vi "AB_Engine_Package_PackedLib.vi"(5 "processed_sourceItems":T1, 7 "application package path":path, 8 "error in (no error)":errorcluster, 10 "destinations":refnum<class "AB_Destination.lvclass">[](array[class]), 11 "internal directory":path) -> (0 "error out":errorcluster, 2 "support dir":path, 3 "dup internal directory":path)   [LabVIEW 2020]
uses:
  <vilib>/AppBuilder/AB_Classes/Destination/AB_Destination.lvclass
  <vilib>/AppBuilder/AB_CopyFiles_Data.ctl
  <vilib>/AppBuilder/AB_Classes/Source/AB_Source_Processed_Info.ctl
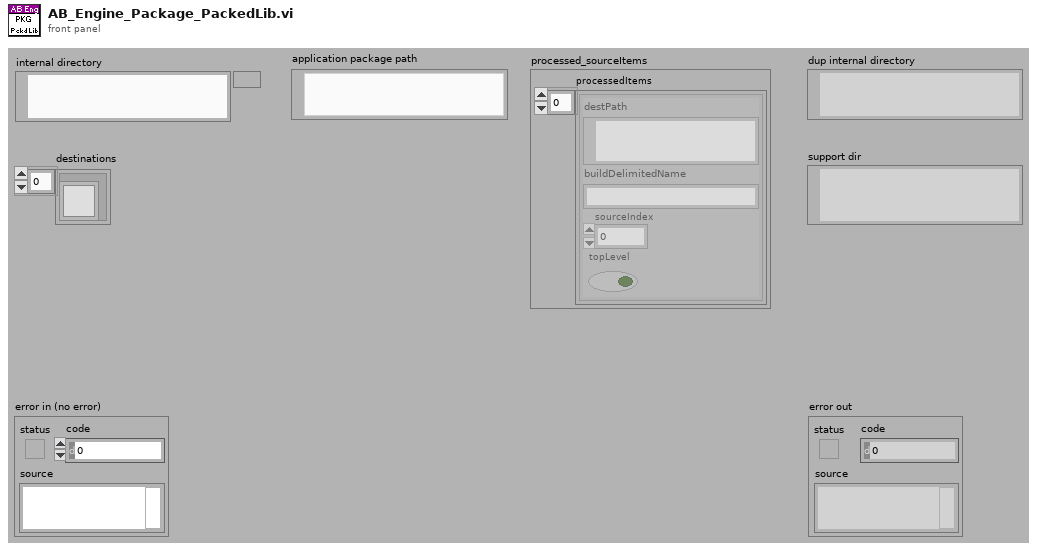
[diagram p1: front panel]
types:
  T1 = typedef "AB_CopyFiles_Data.ctl" = cluster{"processedItems":T2[]}
  T2 = typedef "AB_Source_Processed_Info.ctl" = cluster{"destPath":path, "buildDelimitedName":string, "sourceIndex":i32, "topLevel":bool}
  T3 = enum32{"invalid OS target", "Mac OS", "Windows 3.1", "Windows 95/NT", "Solaris 1", "Solaris 2", "HP-UX", "PowerMAX", "Linux", "Irix", "Rhapsody", "BeOS", "AIX", "OSF1", "VxWorks", "PharLap", "Carbon", "RTX", "Windows x64", "Linux x64", "Mac OS X x64"}
  T4 = typedef "AB_Destination.ctl" = cluster{"destName":string, "path":path, "libraryName":string, "preserveHierarchy":bool, "eng_inBuild":bool, "eng_libraryReference":refnum<vi>, "eng_restictAddToNewLibrary":bool}
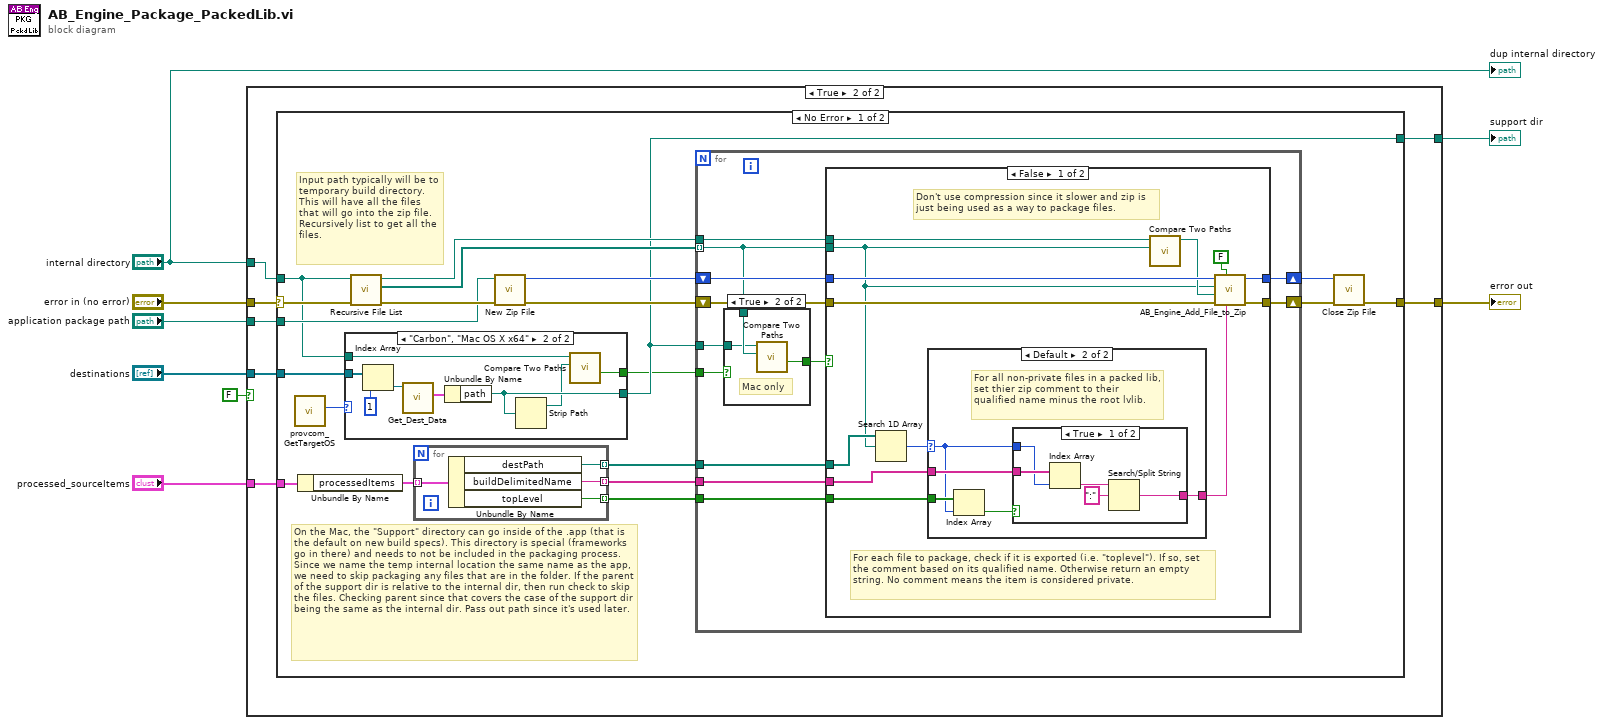
[diagram p0: block diagram]
diagram:
  n1 = case shown="True" FALSE {
    tunnel: [w9 w16] -> w8
    tunnel: "internal directory" -> [_ w15]
    tunnel: "application package path" -> [_ w14]
    tunnel: "error in (no error)" -> [w9 w13]
    tunnel: "destinations" -> [_ w12]
    tunnel: [_ w11] -> w4
    tunnel: "processed_sourceItems" -> [_ w10]
    frame False {
    }
    frame True {
      n2 = case shown="No Error" w13 {
        selector: w13 -> [w27 w89]
        tunnel: [w36 w89] -> w16
        tunnel: w15 -> [w22 _]
        tunnel: w14 -> [w28 _]
        tunnel: w12 -> [w24 _]
        tunnel: [w25 _] -> w11
        tunnel: w10 -> [w20 _]
        frame No Error {
          # "On the Mac, the \"Support\" directory can go inside of the .app (that is the default on new build specs). This directory is special (frameworks go in there) and needs to not be included in the packaging process. Since we name the temp internal location the same name as the app, we need to skip packaging any files that are in the folder. If the parent of the support dir is relative to the internal dir, then run check to skip the files. Checking parent since that covers the case of the support dir being the same as the internal dir. Pass out path since it's used later."
          # "Input path typically will be to temporary build directory. This will have all the files that will go into the zip file. Recursively list to get all the files."
          n3 = call <resource>:"provcom_GetTargetOS.vi"() -> ("App.TargetOS"=w23:T3)  [unwired: 11 out]
          n4 = Unbundle By Name(w20) -> ("processedItems"=w19:T2[])
          n5 = case shown="\"Carbon\", \"Mac OS X x64\"" w23 {
            tunnel: w24 -> [_ w41]
            tunnel: [_ w40] -> w25
            tunnel: w22 -> [_ w39]
            tunnel: [_ w37] -> w21
            frame Default {
            }
            frame "Carbon", "Mac OS X x64" {
              n6 = Index Array(array=w41, index=1) -> (element=w44:refnum<class "AB_Destination.lvclass">)
              n7 = call <vilib>:"Get_Dest_Data.vi"("Class in"=w44) -> ("destName"=w43:T4)  [unwired: 1 in, 9 out]
              n8 = Unbundle By Name(w43) -> ("path"=w40:path)
              n9 = Strip Path(path=w40) -> (stripped path=w38:path)  [unwired: 1 out]
              n10 = call <vilib>:"Compare Two Paths.vi"("Path 2"=w38, "Path 1"=w39) -> ("Path 2 Relative to Path 1?"=w37:bool)  [unwired: 1 in, 8 out]
            }
          }
          n11 = call <vilib>:"Recursive File List.vi"("error in (no error)"=w27, "Folder Path"=w22) -> ("error out"=w29:errorcluster, "All Files in Dir"=w31:path[], "dup Folder Path"=w30:path)  [unwired: 1 in, 6 out]
          n12 = for {
            tunnel: [w46] -> w26 mode=indexing
            tunnel: w19 -> [w48] mode=indexing
            tunnel: [w47] -> w18 mode=indexing
            tunnel: [w45] -> w17 mode=indexing
            n13 = Unbundle By Name(w48) -> ("destPath"=w47:path, "buildDelimitedName"=w46:string, "topLevel"=w45:bool)
          }
          n14 = call <vilib>:"New Zip File.vi"("error in (no error)"=w29, "target"=w28) -> ("error out"=w32:errorcluster, "zip file out"=w35:i64)  [unwired: 1 in, 3 out]
          n15 = for {
            shift-right: [w59] -> w34
            shift-left: w35 -> [w60]
            shift-right: [w58] -> w33
            shift-left: w32 -> [w57]
            tunnel: w31 -> [w55] mode=indexing
            tunnel: w30 -> [w56]
            tunnel: w25 -> [w54]
            tunnel: w18 -> [w52]
            tunnel: w26 -> [w51]
            tunnel: w21 -> [w50]
            tunnel: w17 -> [w49]
            n16 = case shown="True" w50 {
              tunnel: w55 -> [_ w63]
              tunnel: w54 -> [_ w62]
              tunnel: [_ w61] -> w53
              frame False {
              }
              frame True {
                # "Mac only"
                n17 = call <vilib>:"Compare Two Paths.vi"("Path 2"=w63, "Path 1"=w62) -> ("Path 2 Relative to Path 1?"=w61:bool)  [unwired: 1 in, 8 out]
              }
            }
            n18 = case shown="False" w53 {
              tunnel: w60 -> [w76 w87]
              tunnel: [w75 w87] -> w59
              tunnel: [w74 w88] -> w58
              tunnel: w57 -> [w73 w88]
              tunnel: w56 -> [w72 _]
              tunnel: w55 -> [w66 _]
              tunnel: w52 -> [w68 _]
              tunnel: w51 -> [w67 _]
              tunnel: w49 -> [w65 _]
              frame False {
                # "For each file to package, check if it is exported (i.e. \"toplevel\"). If so, set the comment based on its qualified name. Otherwise return an empty string. No comment means the item is considered private."
                # "Don't use compression since it slower and zip is just being used as a way to package files."
                n19 = Search 1D Array(1D array=w68, element=w66) -> (index of element=w64:i32)  [unwired: 1 out]
                n20 = case shown="Default" w64 {
                  selector: w64 -> [_ w78]
                  tunnel: [_ w81] -> w69
                  tunnel: w67 -> [_ w80]
                  tunnel: w65 -> [_ w79]
                  frame -1 {
                  }
                  frame Default {
                    # "For all non-private files in a packed lib, set thier zip comment to their qualified name minus the root lvlib."
                    n21 = Index Array(array=w79, index=w78) -> (element=w77:bool)
                    n22 = case shown="True" w77 {
                      tunnel: [w83 _] -> w81
                      tunnel: w80 -> [w86 _]
                      tunnel: w78 -> [w82 _]
                      frame True {
                        n23 = Index Array(array=w86, index=w82) -> (element=w85:string)
                        n24 = Search/Split String(string=w85, search string/char (-)=":" ("regular expression")) -> (match + rest of string=w83:string)  [unwired: 1 in, 2 out]
                      }
                      frame False {
                      }
                    }
                  }
                }
                n25 = call <vilib>:"Compare Two Paths.vi"("Path 2"=w66, "Path 1"=w72) -> ("Relative Path from 1 to 2"=w71:path)  [unwired: 1 in, 8 out]
                n26 = call <vilib>:"AB_Engine_Add_File_to_Zip.vi"("Comment"=w69, "Compress (T)"=FALSE, "error in (no error)"=w73, "destination path in zip"=w71, "source file path"=w66, "zip file in"=w76) -> ("error out"=w74:errorcluster, "zip file out"=w75:i64)  [unwired: 4 out]
              }
              frame True {
              }
            }
          }
          n27 = call <vilib>:"Close Zip File.vi"("error in (no error)"=w33, "zip file in"=w34) -> ("error out"=w36:errorcluster)  [unwired: 1 in, 4 out]
        }
        frame Error {
        }
      }
    }
  }
  "error out" <- w8
  "support dir" <- w4
  "dup internal directory" <- "internal directory"
